vi "Build_Asylum_GetRange.vi"(8 "error in (no error)":errorcluster, 11 "parameterName":string) -> (0 "error out":errorcluster, 3 "Command":string)   [LabVIEW 2019]
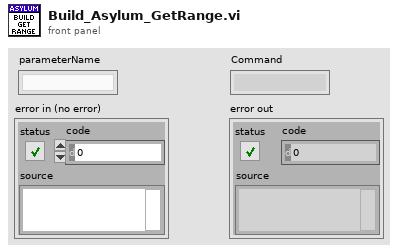
[diagram p1: front panel]
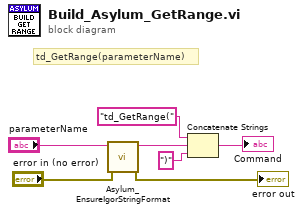
[diagram p0: block diagram]
diagram:
  # "td_GetRange(parameterName)"
  n1 = call "Asylum_EnsureIgorStringFormat.vi"("error in (no error)"="error in (no error)", "Value"="parameterName") -> ("error out"=→"error out":errorcluster, "Value"=w5:string)  [unwired: 8 in]
  n2 = Concatenate Strings("td_GetRange(" ("string"), w5, ")" ("string")) -> (→"Command":string)
